vi "testRead.vi"() -> ()   [LabVIEW 2015]
uses:
  Downloads/Get.GRIP.Data/GRIP Contours Report.ctl
  <vilib>/Rock Robotics/Network Tables/NT Read Numeric Array.vi
  <vilib>/Rock Robotics/Network Tables/NT Read Number.vi
panel:
  out "Connection Count":i32
  out "Connected":bool
  in  "error in (no error)":errorcluster
  out "error out":errorcluster
  out "ContoursReport":T1[](array[typedef])
  out "FPS":dbl
  out "x+y":i32
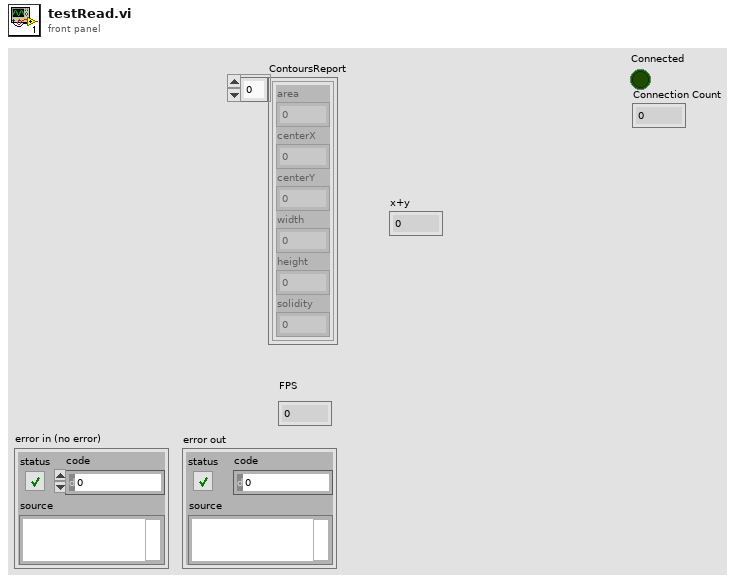
[diagram p1: front panel]
types:
  T1 = typedef "GRIP Contours Report.ctl" = cluster{"area":dbl, "centerX":dbl, "centerY":dbl, "width":dbl, "height":dbl, "solidity":dbl}
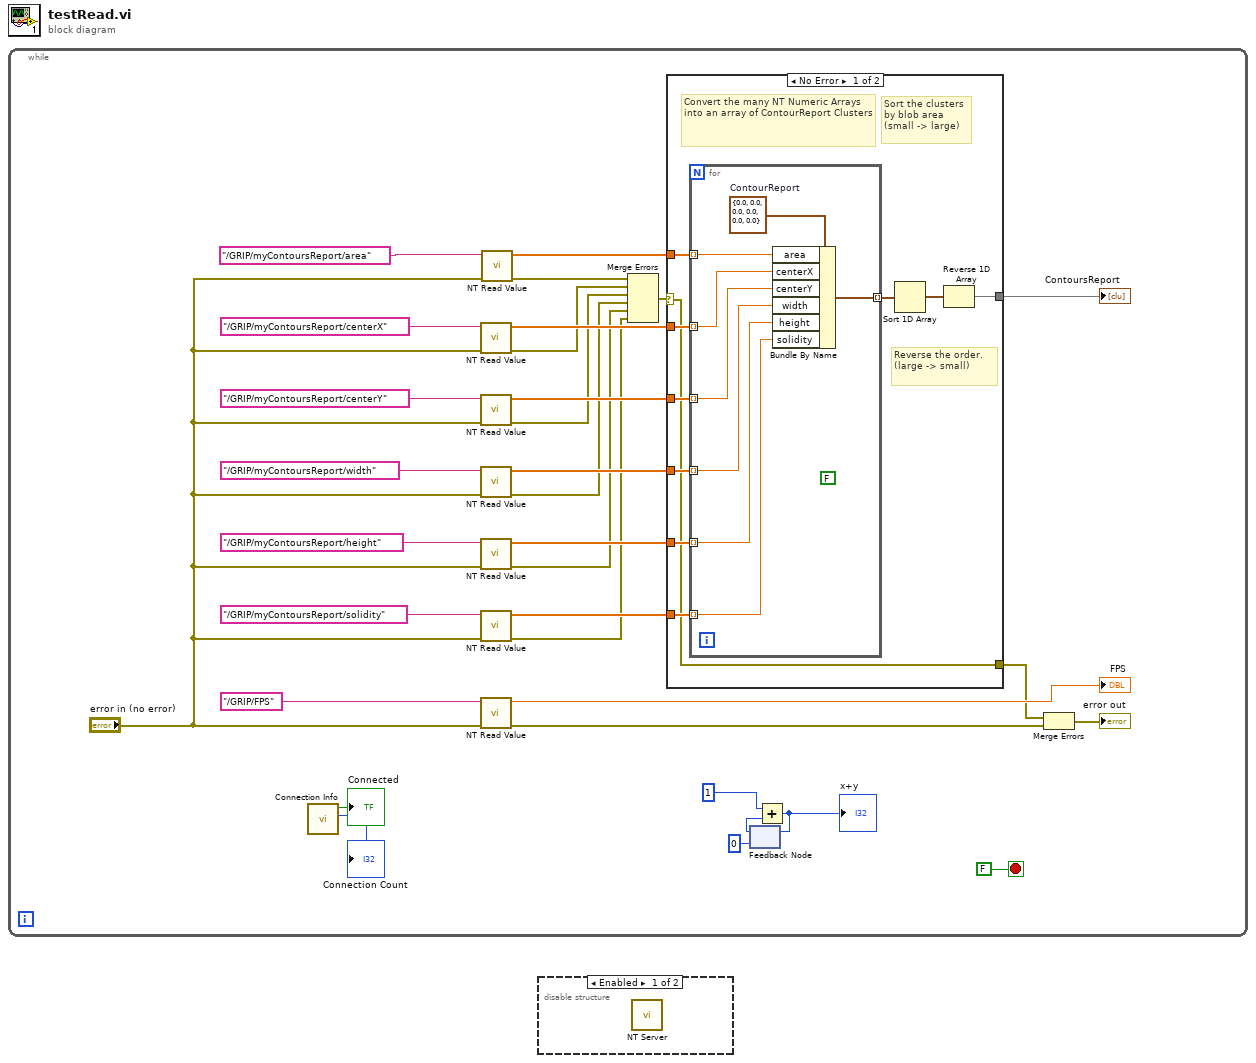
[diagram p0: block diagram]
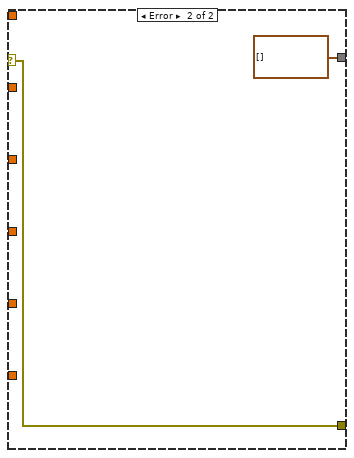
[diagram p3: hidden frame]
diagram:
  n1 = while {
    stop <- FALSE stop-if-true
    (unwired) FALSE
    n2 = call <vilib>:"Connection Info.vi"() -> ("Connection Count"=→"Connection Count":i32, "Connected"=→"Connected":bool)  [unwired: 10 in]
    n3 = call-poly <vilib>:"NT Read Value.vi"("error in"="error in (no error)", "Name"="/GRIP/myContoursReport/centerX") -> ("error out"=w9:errorcluster, "Numeric Array"=w17:dbl[])  [unwired: 8 in]
    n4 = call-poly <vilib>:"NT Read Value.vi"("error in"="error in (no error)", "Name"="/GRIP/myContoursReport/centerY") -> ("error out"=w10:errorcluster, "Numeric Array"=w18:dbl[])  [unwired: 8 in]
    n5 = call-poly <vilib>:"NT Read Value.vi"("error in"="error in (no error)", "Name"="/GRIP/myContoursReport/width") -> ("error out"=w11:errorcluster, "Numeric Array"=w19:dbl[])  [unwired: 8 in]
    n6 = call-poly <vilib>:"NT Read Value.vi"("error in"="error in (no error)", "Name"="/GRIP/myContoursReport/height") -> ("error out"=w12:errorcluster, "Numeric Array"=w20:dbl[])  [unwired: 8 in]
    n7 = call-poly <vilib>:"NT Read Value.vi"("error in"="error in (no error)", "Name"="/GRIP/myContoursReport/solidity") -> ("error out"=w13:errorcluster, "Numeric Array"=w21:dbl[])  [unwired: 8 in]
    n8 = call-poly <vilib>:"NT Read Value.vi"("error in"="error in (no error)", "Name"="/GRIP/FPS" ("Variable")) -> ("error out"=w6:errorcluster, "Numeric"=→"FPS":dbl)  [unwired: 8 in]
    n9 = call-poly <vilib>:"NT Read Value.vi"("error in"="error in (no error)", "Name"="/GRIP/myContoursReport/area") -> ("error out"=w14:errorcluster, "Numeric Array"=w16:dbl[])  [unwired: 8 in]
    n10 = Merge Errors(w14, w9, w10, w11, w12, w13) -> (w8:errorcluster)
    n11 = case shown="No Error" w8 {
      selector: w8 -> [w34 w52]
      tunnel: w21 -> [w43 _]
      tunnel: w20 -> [w42 _]
      tunnel: w19 -> [w41 _]
      tunnel: w18 -> [w40 _]
      tunnel: w17 -> [w39 _]
      tunnel: w16 -> [w38 _]
      tunnel: [w35 T1[] []] -> w15
      tunnel: [w34 w52] -> w7
      frame No Error {
        # "Reverse the order.\n(large -> small)"
        # "Sort the clusters by blob area\n(small -> large)"
        # "Convert the many NT Numeric Arrays into an array of ContourReport Clusters"
        n12 = for {
          tunnel: w43 -> [w49] mode=indexing
          tunnel: w42 -> [w48] mode=indexing
          tunnel: w41 -> [w47] mode=indexing
          tunnel: w40 -> [w46] mode=indexing
          tunnel: w39 -> [w45] mode=indexing
          tunnel: w38 -> [w50] mode=indexing
          tunnel: [w44] -> w37 mode=indexing
          w51 = T1 {"area"=0.0, "centerX"=0.0, "centerY"=0.0, "width"=0.0, "height"=0.0, "solidity"=0.0}  # ContourReport
          n13 = Bundle By Name(cluster=w51, "area"=w50, "centerX"=w45, "centerY"=w46, "width"=w47, "height"=w48, "solidity"=w49) -> (w44:T1)
        }
        n14 = Sort 1D Array(array=w37) -> (sorted array=w36:T1[])
        n15 = Reverse 1D Array(array=w36) -> (reversed array=w35:T1[])
      }
      frame Error {
      }
    }
    "ContoursReport" <- w15
    n16 = feedback #1(0) -> (w31:i32)
    n17 = Add(x=1, y=w31) -> (x+y=w32:i32)
    "x+y" <- w32
    n18 = feedback-in #1(w32) -> ()
    n19 = Merge Errors(w7, w6) -> (→"error out":errorcluster)
  }
  n20 = disable-structure shown="Enabled" {
    frame Enabled {
      n21 = call <vilib>:"NT Server.vi"() -> ()  [unwired: 12 in]
    }
    frame Disabled {
    }
  }
